vi "DrawCityTest.vi"() -> ()   [LabVIEW 2025]
panel:
  in  "path to PNG file":path
  out "new picture":picture
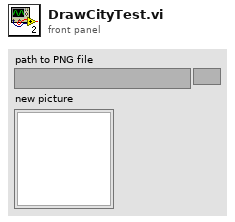
[diagram p1: front panel]
types:
  T1 = cluster{"left":i16, "top":i16, "right":i16, "bottom":i16}
  T2 = typedef "imagedata.ctl" = cluster{"image type":i32, "image depth":i32, "image":u8[], "mask":u8[], "colors":u32[], "Rectangle":cluster{"left":i16, "top":i16, "right":i16, "bottom":i16}}
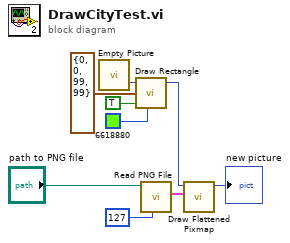
[diagram p0: block diagram]
diagram:
  n1 = call "Empty Picture"() -> ("empty picture"=w8:picture)
  n2 = call <vilib>:"Draw Rectangle.vi"("picture"=w8, "rect"=T1 {"left"=0, "top"=0, "right"=99, "bottom"=99}, "fill?(F)"=TRUE, "color(black)"=u32 6618880) -> ("new picture"=w2:picture)  [unwired: 5 in]
  n3 = call <vilib>:"Read PNG File.vi"("Transparency Thresh"=u8 127, "path to PNG file"="path to PNG file") -> ("image data"=w4:T2)  [unwired: 7 in, 2 out]
  n4 = call <vilib>:"Draw Flattened Pixmap.vi"("image data"=w4, "picture"=w2) -> ("new picture"=→"new picture":picture)  [unwired: 7 in]
